vi "Create Y Rotation Matrix.vi"(11 "Theta (°)":sgl) -> (3 "Rotation Y Matrix":sgl[][](array[numeric]))   [LabVIEW 2020, in "3D.lvlib"]
uses:
  Libraries/3D/3D.lvlib
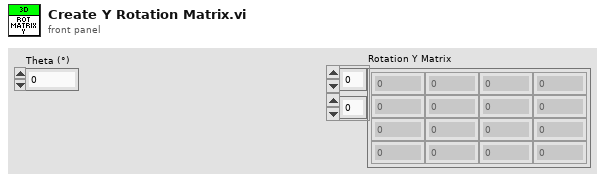
[diagram p1: front panel]
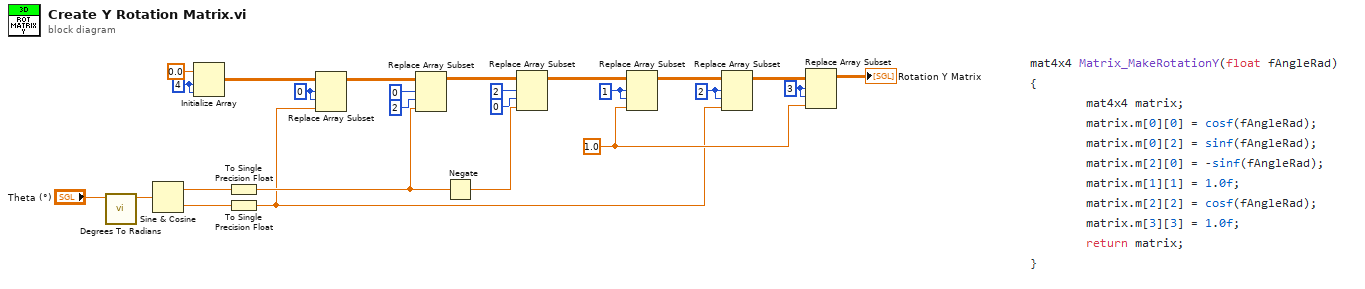
[diagram p0: block diagram]
diagram:
  w4 = sgl 1.0 ("new element/subarray")
  w22 = 3 ("index (row)")
  w20 = 2 ("index (row)")
  w19 = 1 ("index (row)")
  w10 = 0 ("index (row)")
  w9 = 4 ("dimension size")
  n1 = call "Degrees To Radians.vi"("Angle (°)"="Theta (°)") -> ("Angle (rad)"=w1:sgl)  [unwired: 10 in]
  n2 = Sine & Cosine(0:w1) -> (1:w7:sgl, 2:w5:sgl)
  n3 = Initialize Array(sgl 0.0 ("element"), w9, w9) -> (w25:sgl[][])
  n4 = To Single Precision Float(number=w7) -> (single precision float=w6:sgl)
  n5 = To Single Precision Float(number=w5) -> (single precision float=w3:sgl)
  n6 = Replace Array Subset(array=w25, new element=w3, index (row)=w10, index (col)=w10) -> (w11:sgl[][])
  n7 = Replace Array Subset(array=w11, new element=w6, index (row)=0, index (col)=2 ("disabled index (col)")) -> (w14:sgl[][])
  n8 = Negate(x=w6) -> (-x=w23:sgl)
  n9 = Replace Array Subset(array=w14, new element=w23, index (row)=2, index (col)=0 ("index (row)")) -> (w15:sgl[][])
  n10 = Replace Array Subset(array=w15, new element=w4, index (row)=w19, index (col)=w19) -> (w16:sgl[][])
  n11 = Replace Array Subset(array=w16, new element=w3, index (row)=w20, index (col)=w20) -> (w21:sgl[][])
  n12 = Replace Array Subset(array=w21, new element=w4, index (row)=w22, index (col)=w22) -> (→"Rotation Y Matrix":sgl[][])
